vi "raptor_set_en_face_depth.vi"(8 "error in (no error)":errorcluster, 11 "Depth":dbl) -> (0 "error out":errorcluster)   [LabVIEW 2016]
doc: "Raptor: Change the en face display depth without re-initialising."
uses:
  typedef/raptor_message.ctl
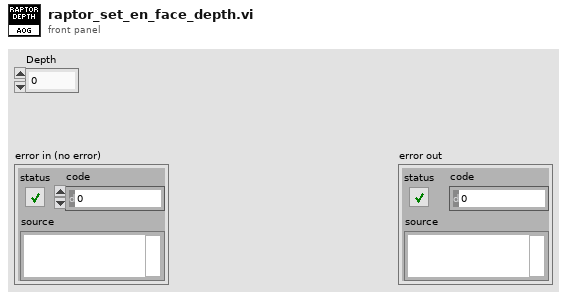
[diagram p1: front panel]
types:
  T1 = typedef "raptor_message.ctl" = cluster{"Message":enum16{"start", "stop", "initialise", "shutdown", "end scan", "new scan", "set depth"}, "Data":variant}
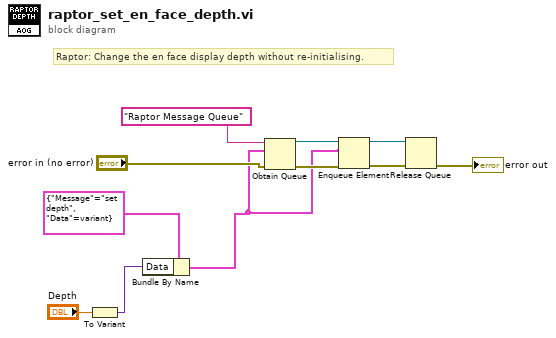
[diagram p0: block diagram]
diagram:
  # "Raptor: Change the en face display depth without re-initialising."
  n1 = To Variant(anything="Depth") -> (Variant=w1:variant)
  n2 = Bundle By Name(cluster=T1 {"Message"=enum."set depth", "Data"=variant} ("Cluster"), "Data"=w1) -> (w3:T1)
  n3 = Obtain Queue(name (unnamed)="Raptor Message Queue", element data type=w3, error in (no error)="error in (no error)") -> (queue out=w10:refnum<queue>, error out=w6:errorcluster)  [unwired: 2 in, 1 out]
  n4 = Enqueue Element(queue=w10, element=w3, error in (no error)=w6) -> (queue out=w9:refnum<queue>, error out=w7:errorcluster)  [unwired: 1 in, 1 out]
  n5 = Release Queue(queue=w9, error in (no error)=w7) -> (error out=→"error out":errorcluster)  [unwired: 1 in, 2 out]
